vi "USB2XXXIIC24C02.vi"() -> ()   [LabVIEW 2010]
uses:
  PublicFiles/usb_device/USB2XXX.dll
panel:
  out "Read Data(Hex)":string
  in  "Read Data Count":i32=8
  in  "Reg Addr(Hex)":u8 format="%x"
  in  "Slave Addr(Hex)":i16=80 format="%x"
  in  "Write Data(Hex)":string="11 22 33 44 55 66 77 88"
  in  "pConfig":T1
  in  "Channel Index":i32(ring) items=["CH0", "CH1", "CH2", "CH3", "CH4", "CH5", "CH6", "CH7"]
  in  "Device Index":i32(ring) items=["0", "1", "2", "3", "4", "5"]
  out "Flag(T:Write;F:Read)":bool=TRUE
  in  "stop":bool
  in  "Read":bool
  in  "Write":bool
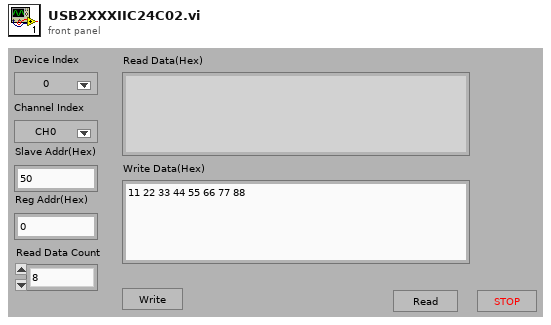
[diagram p1: front panel]
types:
  T1 = cluster{"ClockSpeedHz":u32, "OwnAddr":u16, "Master":u8, "AddrBits":u8, "EnablePu":u8}
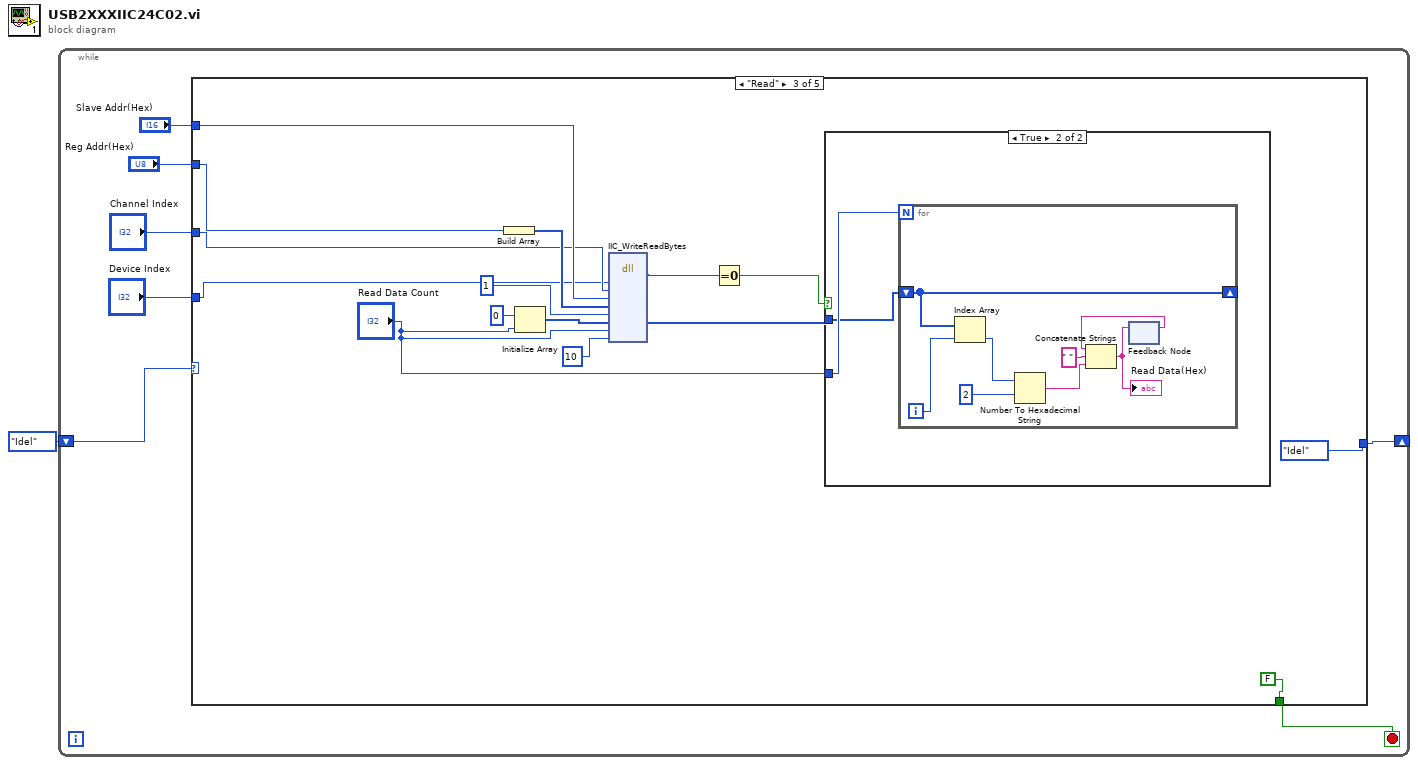
[diagram p0: block diagram]
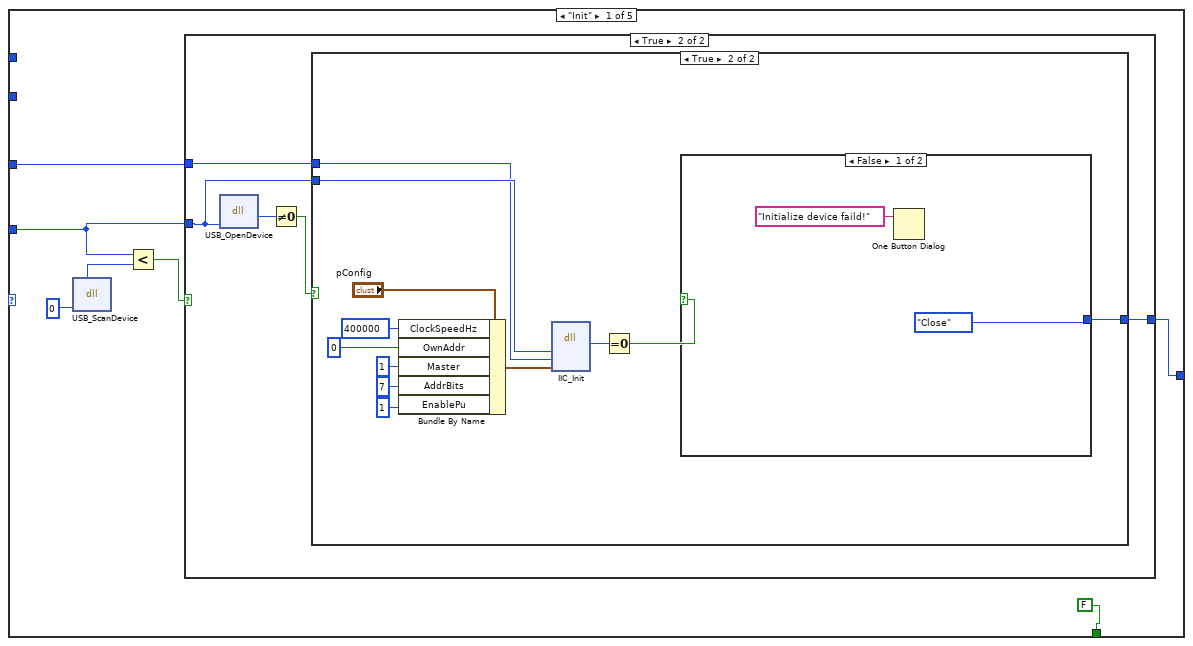
[diagram p2: hidden frame]
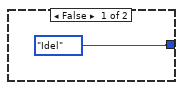
[diagram p3: hidden frame]
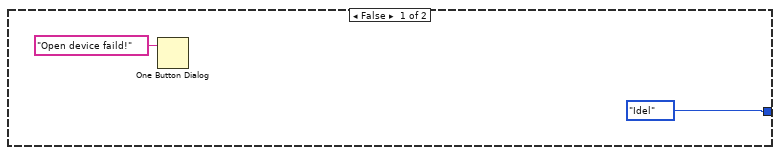
[diagram p4: hidden frame]
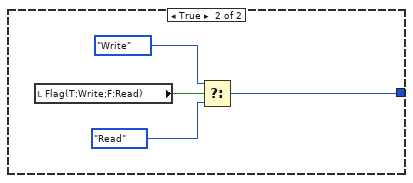
[diagram p5: hidden frame]
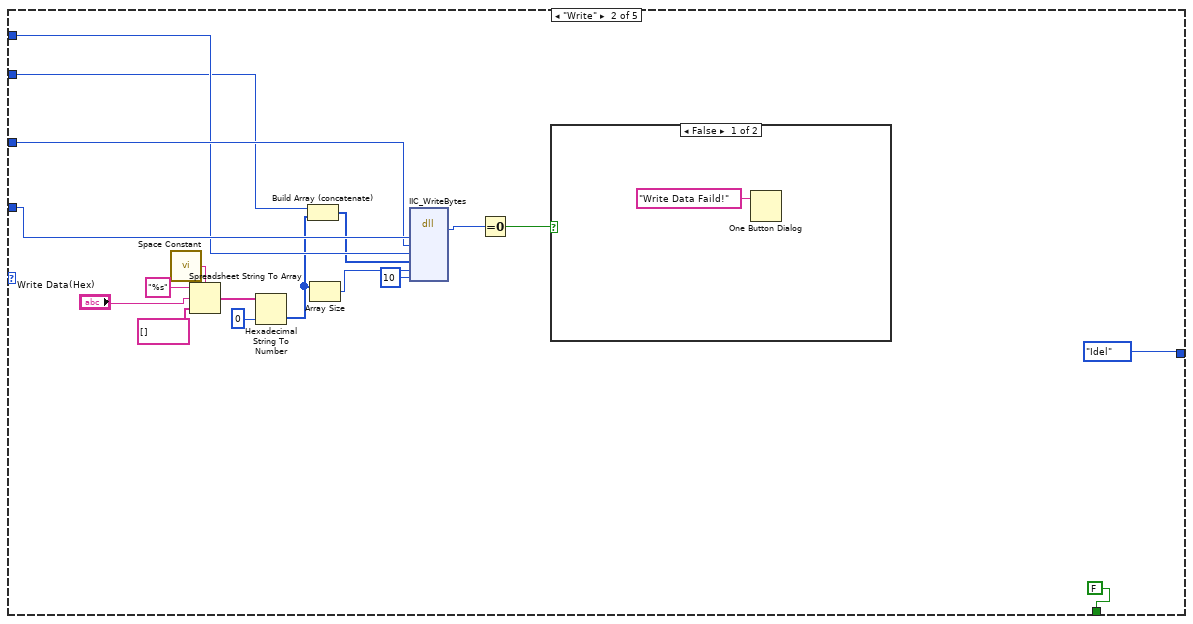
[diagram p6: hidden frame]
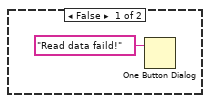
[diagram p8: hidden frame]
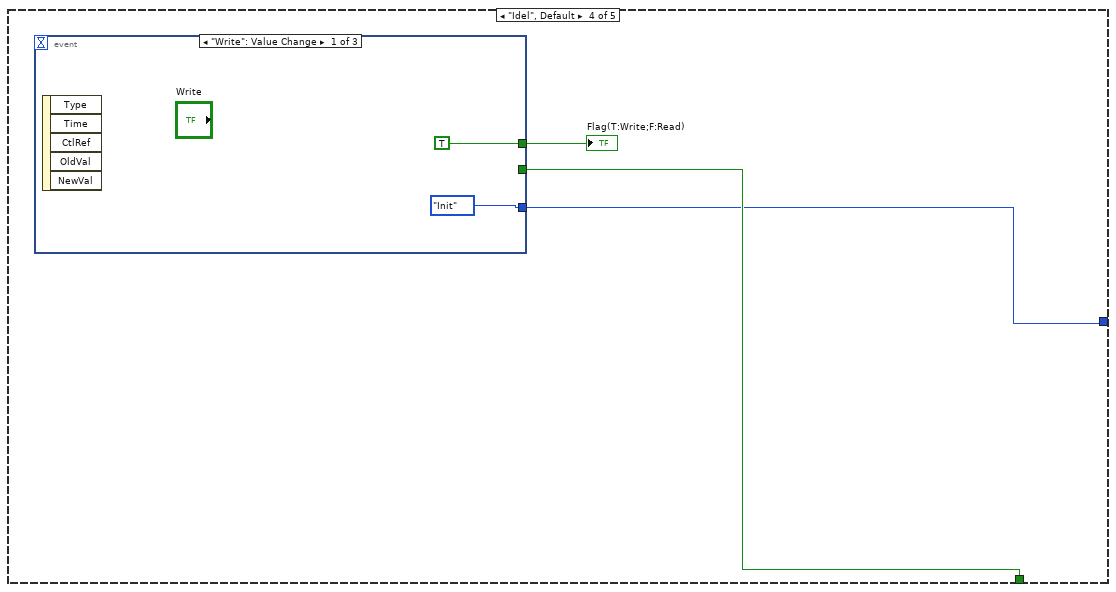
[diagram p9: hidden frame]
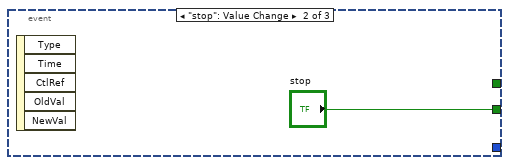
[diagram p10: hidden frame]
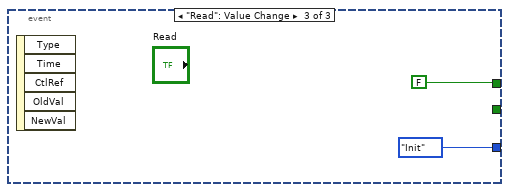
[diagram p11: hidden frame]
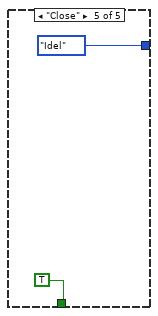
[diagram p12: hidden frame]
diagram:
  n1 = while {
    shift-right: [w7] -> _
    shift-left: enum16{"Init", "Write", "Read", "Idel", "Close"}."Idel" ("Enum") -> [w8]
    stop <- w2 stop-if-true
    n2 = case shown="\"Read\"" w8 {
      tunnel: [w12 enum16{"Init", "Write", "Read", "Idel", "Close"}."Idel" ("Enum") enum16{"Init", "Write", "Read", "Idel", "Close"}."Idel" ("Enum") w87 enum16{"Init", "Write", "Read", "Idel", "Close"}."Idel" ("Enum")] -> w7
      tunnel: "Device Index" -> [w11 w53 w67 _ _]
      tunnel: "Channel Index" -> [w10 w52 w68 _ _]
      tunnel: "Slave Addr(Hex)" -> [_ w46 w69 _ _]
      tunnel: "Reg Addr(Hex)" -> [_ w45 w72 _ _]
      tunnel: [FALSE FALSE FALSE w88 TRUE] -> w2
      frame "Init" {
        n3 = dll-call lib="F:/OtherWork/STM32/USB2XXX_Example/trunk/Labview/PublicFiles/usb_device/USB2XXX.*" fn="USB_ScanDevice"("pDevNum"=0) -> (w14:i32)  [unwired: 4 in, 2 out]
        n4 = Less?(x=w11, y=w14) -> (x < y?=w13:bool)
        n5 = case shown="True" w13 {
          tunnel: w11 -> [_ w18]
          tunnel: w10 -> [_ w19]
          tunnel: [enum16{"Init", "Write", "Read", "Idel", "Close"}."Idel" ("Enum") w17] -> w12
          frame False {
          }
          frame True {
            n6 = dll-call lib="F:/OtherWork/STM32/USB2XXX_Example/trunk/Labview/PublicFiles/usb_device/USB2XXX.*" fn="USB_OpenDevice"("DevIndex"=w18) -> (w21:u8)  [unwired: 4 in, 2 out]
            n7 = Not Equal To 0?(x=w21) -> (x != 0?=w20:bool)
            n8 = case shown="True" w20 {
              tunnel: w19 -> [_ w27]
              tunnel: w18 -> [_ w28]
              tunnel: [enum16{"Init", "Write", "Read", "Idel", "Close"}."Idel" ("Enum") w24] -> w17
              frame False {
                n9 = One Button Dialog(message="Open device faild!") -> ()  [unwired: 1 in, 1 out]
              }
              frame True {
                n10 = Bundle By Name(cluster="pConfig", "ClockSpeedHz"=u32 400000, "OwnAddr"=u16 0, "Master"=u8 1, "AddrBits"=u8 7, "EnablePu"=u8 1) -> (w34:T1)
                n11 = dll-call lib="F:/OtherWork/STM32/USB2XXX_Example/trunk/Labview/PublicFiles/usb_device/USB2XXX.*" fn="IIC_Init"("DevIndex"=w28, "IICIndex"=w27, "pConfig"=w34) -> (w26:i32)  [unwired: 6 in, 2 out]
                n12 = Equal To 0?(x=w26) -> (x = 0?=w25:bool)
                n13 = case shown="False" w25 {
                  tunnel: [enum16{"Init", "Write", "Read", "Idel", "Close"}."Close" ("Enum") w38] -> w24
                  frame False {
                    n14 = One Button Dialog(message="Initialize device faild!") -> ()  [unwired: 1 in, 1 out]
                  }
                  frame True {
                    n15 = local read "Flag(T:Write;F:Read)"() -> (w41:bool)
                    n16 = Select(t=enum16{"Init", "Write", "Read", "Idel", "Close"}."Write" ("Enum"), s=w41, f=enum16{"Init", "Write", "Read", "Idel", "Close"}."Read" ("Enum")) -> (s? t:f=w38:enum16{"Init", "Write", "Read", "Idel", "Close"})
                  }
                }
              }
            }
          }
        }
      }
      frame "Write" {
        n17 = call <vilib>:"Space Constant.vi"() -> ("String"=w55:string)
        n18 = Spreadsheet String To Array(delimiter (Tab)=w55, format string="%s", spreadsheet string="Write Data(Hex)", array type (2D Dbl)=string[] []) -> (array=w58:string[])
        n19 = Hexadecimal String To Number(string=w58, default (0uL)=u8 0 ("default (0 U32)")) -> (number=w44:u8[])  [unwired: 1 in, 1 out]
        n20 = Build Array (concatenate)(w45, w44) -> (w43:u8[])
        n21 = Array Size(array=w44) -> (size(s)=w51:i32)
        n22 = dll-call lib="F:/OtherWork/STM32/USB2XXX_Example/trunk/Labview/PublicFiles/usb_device/USB2XXX.*" fn="IIC_WriteBytes"("DevIndex"=w53, "IICIndex"=w52, "SlaveAddr"=w46, "pWriteData"=w43, "WriteLen"=w51, "TimeOutMs"=10) -> (w49:i32)  [unwired: 9 in, 2 out]
        n23 = Equal To 0?(x=w49) -> (x = 0?=w48:bool)
        n24 = case shown="False" w48 {
          frame False {
            n25 = One Button Dialog(message="Write Data Faild!") -> ()  [unwired: 1 in, 1 out]
          }
          frame True {
          }
        }
      }
      frame "Read" {
        n26 = Build Array(w72) -> (w70:u8[])
        n27 = Initialize Array(u8 0 ("element"), "Read Data Count") -> (w73:u8[])
        n28 = dll-call lib="F:/OtherWork/STM32/USB2XXX_Example/trunk/Labview/PublicFiles/usb_device/USB2XXX.*" fn="IIC_WriteReadBytes"("DevIndex"=w67, "IICIndex"=w68, "SlaveAddr"=w69, "pWriteData"=w70, "WriteLen"=1 ("dimension size"), "pReadData"=w73, "ReadLen"="Read Data Count", "TimeOutMs"=10) -> (w66:i32, "pReadData"=w62:u8[])  [unwired: 10 in, 2 out]
        n29 = Equal To 0?(x=w66) -> (x = 0?=w65:bool)
        n30 = case shown="True" w65 {
          tunnel: "Read Data Count" -> [_ w78]
          tunnel: w62 -> [_ w77]
          frame False {
            n31 = One Button Dialog(message="Read data faild!") -> ()  [unwired: 1 in, 1 out]
          }
          frame True {
            n32 = for {
              N: w78 -> [_]
              shift-right: [w79] -> _
              shift-left: w77 -> [w79]
              i -> [w86]
              n33 = Index Array(array=w79, index=w86) -> (element=w85:u8)
              n34 = Number To Hexadecimal String(1:i16 2 ("width (-)"), 2:w85) -> (0:w81:string)
              n35 = feedback #1() -> (w83:string)  [unwired: 1 in]
              n36 = Concatenate Strings(w83, " " ("string"), w81) -> (w80:string)
              "Read Data(Hex)" <- w80
              n37 = feedback-in #1(w80) -> ()
            }
          }
        }
      }
      frame "Idel", Default {
        n38 = event shown="[0] \"Write\": Value Change" {
          selector: _ -> [_ _ _]
          dyn-events: _ -> [_ _ _]
          timeout: _ -> [_ _ _]
          tunnel: [TRUE _ FALSE] -> w89
          tunnel: [_ "stop" _] -> w88
          tunnel: [enum16{"Init", "Write", "Read", "Idel", "Close"}."Init" ("Enum") _ enum16{"Init", "Write", "Read", "Idel", "Close"}."Init" ("Enum")] -> w87
          event "Write": Value Change {
            n39 = event-data() -> ()  [unwired: 1 in, 5 out]
          }
          event "stop": Value Change {
            n40 = event-data() -> ()  [unwired: 1 in, 5 out]
          }
          event "Read": Value Change {
            n41 = event-data() -> ()  [unwired: 1 in, 5 out]
          }
        }
        "Flag(T:Write;F:Read)" <- w89
      }
      frame "Close" {
      }
    }
  }
